vi "vapor_temp_psat_density.vi"(0 "Vapor Temp [C}":dynamicdata(graph)) -> (1 "Psat Vapor":dbl, 2 "Vapor Density":dbl, 3 "Vapor Density Array":dbl[](array[numeric]))   [LabVIEW 2015]
uses:
  <vilib>/express/express arith-compare/Formula/XNode/ExpressFormulaBlockNode.xnode
  <vilib>/express/express shared/transition.llb/Dynamic To Waveform Array.vi
  <vilib>/express/express arith-compare/Formula/Block/exnFormulaBlock how many pts in the wave.vi
  <vilib>/express/express shared/ex_Modify Signal Name.vi
  <vilib>/express/express shared/transition.llb/Waveform Array To Dynamic.vi
panel:
  in  "Vapor Temp [C]":i32
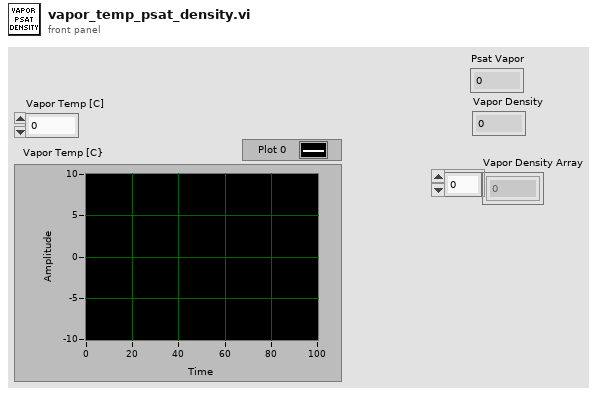
[diagram p1: front panel]
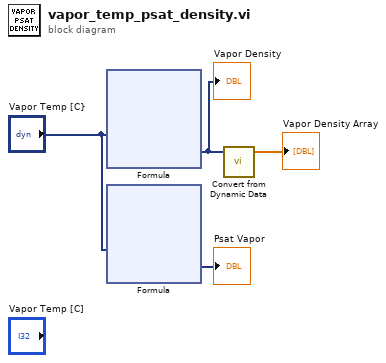
[diagram p0: block diagram]
diagram:
  n1 = xnode "Formula"("T"="Vapor Temp [C}") -> ("Result"=w2:dynamicdata)  [unwired: 1 in, 1 out]
  "Vapor Density" <- w2
  n2 = xnode "Formula"("T"="Vapor Temp [C}") -> ("Result"=→"Psat Vapor":dynamicdata)  [unwired: 1 in, 1 out]
  n3 = call "Convert from Dynamic Data"("Dynamic Data Type"=w2) -> ("Array"=→"Vapor Density Array":dbl[])  [unwired: 3 in]
